vi "Continuous Sound Input.vi"() -> ()   [LabVIEW 2023]
doc: "This VI illustrates how to acquire sound samples continuously from a specified device. It requires the use of a microphone attached to the sound card. You can specify the number of samples to acquire, sample rate, number of channels and a bit rate per sample. The VI also plots the raw data as the acquisition is made."
uses:
  <vilib>/sound2/lvsound2.llb/Sampling Mode.ctl
  <vilib>/sound2/lvsound2.llb/Sound Data Format.ctl
  <vilib>/sound2/lvsound2.llb/Sound Input Read (DBL).vi
panel:
  in  "Device ID":u32 format="%.0x"
  in  "Number of Samples/ch":i32=5000
  out "Raw Data":waveform(dbl)[](graph)
  in  "Stop":bool
  # "Overview: Demonstrates the use of the Sound Input Functions to acquire sound samples continuously with the use of a microphone attached to the sound card.\nRequirements: Microphone\nInstructions:\n1. Specify the Device ID and Number of Samples/ch.\n2. Run the VI.\n3. The VI will continuously acquire samples and plot the raw data to the graph.\n4. Click Stop to stop the VI."
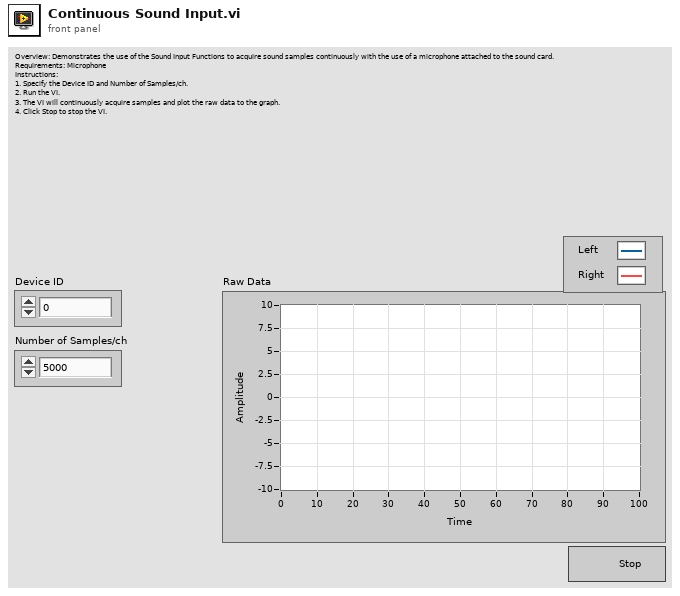
[diagram p1: front panel]
types:
  T1 = typedef "Sound Data Format.ctl" = cluster{"sample rate (S/s)":dbl, "number of channels":i32, "bits per sample":i32}
  T2 = typedef "Sampling Mode.ctl" = i32
  T3 = typedef "Sound Input Task ID.ctl" = u32
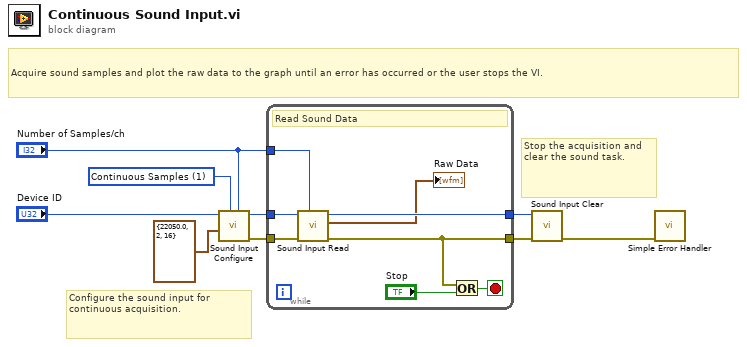
[diagram p0: block diagram]
diagram:
  w4 = T2 1 items=["Finite Samples", "Continuous Samples"] ("sample mode")
  # "Acquire sound samples and plot the raw data to the graph until an error has occurred or the user stops the VI."
  # "Stop the acquisition and clear the sound task."
  # "Configure the sound input for continuous acquisition."
  n1 = call <vilib>:"Sound Input Configure.vi"("number of samples/ch"="Number of Samples/ch", "sample mode"=w4, "sound format"=T1 {"sample rate (S/s)"=22050.0, "number of channels"=2, "bits per sample"=16} ("Sound Format"), "device ID"="Device ID") -> ("error out"=w9:errorcluster, "task ID"=w7:T3)  [unwired: 6 in]
  n2 = while {
    tunnel: w7 -> [w16]
    tunnel: [w15] -> w6
    tunnel: "Number of Samples/ch" -> [w14]
    tunnel: w9 -> [w17]
    tunnel: [w10] -> w5
    stop <- w12 stop-if-true
    # "Read Sound Data"
    n3 = call-poly <vilib>:"Sound Input Read.vi"("number of samples/ch"=w14, "error in (no error)"=w17, "task ID"=w16) -> ("error out"=w10:errorcluster, "data"=→"Raw Data":waveform(dbl)[], "task ID out"=w15:T3)  [unwired: 6 in]
    n4 = Or(x=w10, y="Stop") -> (x .or. y?=w12:bool)
  }
  n5 = call <vilib>:"Sound Input Clear.vi"("error in (no error)"=w5, "task ID"=w6) -> ("error out"=w2:errorcluster)  [unwired: 9 in]
  n6 = call <vilib>:"Simple Error Handler.vi"("error in (no error)"=w2) -> ()  [unwired: 4 in, 5 out]
